vi "Both Gyros.vi"(9 "Set To":dbl format="%#_13g", 10 "Reset":bool, 11 "Enum":T1) -> (3 "Angle":dbl)   [LabVIEW 2014]
uses:
  TypeDefs/SRE Enum.ctl
  <vilib>/Rock Robotics/Network Tables/SD Read Boolean.vi
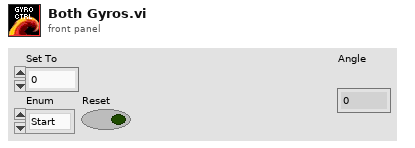
[diagram p1: front panel]
types:
  T1 = typedef "SRE Enum.ctl" = enum16{"Start", "Run", "End"}
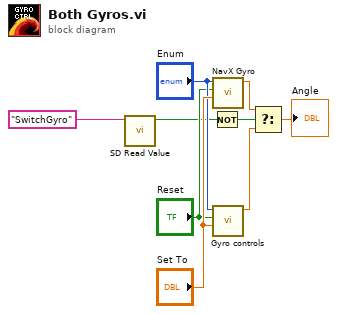
[diagram p0: block diagram]
diagram:
  n1 = call-poly <vilib>:"SD Read Value.vi"("Name"="SwitchGyro") -> ("Boolean"=w3:bool)  [unwired: 8 in, 2 out]
  n2 = Not(x=w3) -> (.not. x?=w2:bool)
  n3 = call "NavX Gyro.vi"("Set To"="Set To", "Reset"="Reset", "Enum"="Enum") -> ("Angle"=w6:dbl)  [unwired: 7 in, 1 out]
  n4 = call "Gyro controls.vi"("Set To"="Set To", "Reset"="Reset", "Enum"="Enum") -> ("Angle"=w5:dbl)  [unwired: 8 in]
  n5 = Select(t=w6, s=w2, f=w5) -> (s? t:f=→"Angle":dbl)
